vi "Launch as Nested Actor.vi"(6 "timeout in ms (-1)":i32=-1, 8 "Error In":errorcluster, 9 "Panel":refnum<class "Panel.lvclass">, 10 "Panel Actor in":refnum<class "Panel Actor.lvclass">, 11 "Caller Actor in":refnum<class "Actor.lvclass">) -> (0 "Error Out":errorcluster, 2 "Actor's Enqueuer":refnum<class "Message Enqueuer.lvclass">, 3 "Caller Actor out":refnum<class "Actor.lvclass">)   [LabVIEW 2023, in "Panel Actor.lvlib" / "Panel Actor.lvclass"]
doc: "Launches a root panel as a nested actor of a non-panel actor.\n\n<B>Caller Actor In:</B> Nested caller Actor \n<B>Panel Actor In:</B> Panel actor to launch as nested actor\n<B>Panel:</B> Panel to use in displaying nested actor\n<B>timeout in ms</B> Time to wait for the panel to initialize\n<B>Error In:</B> Describes error conditions that occur before this node runs.\n\n<B>Caller Actor In:</B> Nested caller Actor \n<B>Actor's Enqueuer:</B> Enqueuer for newly spawned actor\n<B>Error Out:</B> Contains error information.\n----\nPlease see the following web address for additional documentation and tutorial information:\nhttp://www.mooregoodideas.com/mgi-panel-manager/\n\nAuthor: Derek Trepanier\n\nCopyright (c) 2018, Moore Good Ideas, Inc.\n\nAll rights reserved.\n\nRedistribution and use in source and binary forms, with or without modification, are permitted provided that the following conditions are met:\n\n * Redistributions of source code must retain the above copyright notice, this list of conditions and the following disclaimer.\n * Redistributions in binary form must reproduce the above copyright notice, this list of conditions and the following disclaimer in the documentation and/or other materials provided with the distribution.\n * Neither the name of Moore Good Ideas, Inc. nor the names of its contributors may be used to endorse or promote products derived from this software without specific prior written permission.\n\nTHIS SOFTWARE IS PROVIDED BY THE COPYRIGHT HOLDERS AND CONTRIBUTORS \"AS IS\" AND ANY EXPRESS OR IMPLIED WARRANTIES, INCLUDING, BUT NOT LIMITED TO, THE IMPLIED WARRANTIES OF MERCHANTABILITY AND FITNESS FOR A PARTICULAR PURPOSE ARE DISCLAIMED. IN NO EVENT SHALL THE COPYRIGHT OWNER OR CONTRIBUTORS BE LIABLE FOR ANY DIRECT, INDIRECT, INCIDENTAL, SPECIAL, EXEMPLARY, OR CONSEQUENTIAL DAMAGES (INCLUDING, BUT NOT LIMITED TO, PROCUREMENT OF SUBSTITUTE GOODS OR SERVICES; LOSS OF USE, DATA, OR PROFITS; OR BUSINESS INTERRUPTION) HOWEVER CAUSED AND ON ANY THEORY OF LIABILITY, WHETHER IN CONTRACT, STRICT LIABILITY, OR TORT (INCLUDING NEGLIGENCE OR OTHERWISE) ARISING IN ANY WAY OUT OF THE USE OF THIS SOFTWARE, EVEN IF ADVISED OF THE POSSIBILITY OF SUCH DAMAGE."
uses:
  Library/Panel Actor.lvclass
  Panel/Panel/Panel.lvclass
  builds/Framework/Actor Framework.lvlibp/1abvi3w/vi.lib/ActorFramework/Message Enqueuer/Message Enqueuer.lvclass
  builds/Framework/Actor Framework.lvlibp/1abvi3w/vi.lib/ActorFramework/Actor/Actor.lvclass
  Panel/Panel/Panel.lvclass/Panel.ctl
  Library/Panel Actor.lvclass/Panel Actor.ctl
  Panel/Init Waiter/Init Waiter.vi
  Panel/Init Waiter/Init Waiter.lvclass
  C:/Users/Public/Documents/Development/builds/Framework/Actor Framework.lvlibp/1abvi3w/vi.lib/ActorFramework/Actor/Actor.lvclass
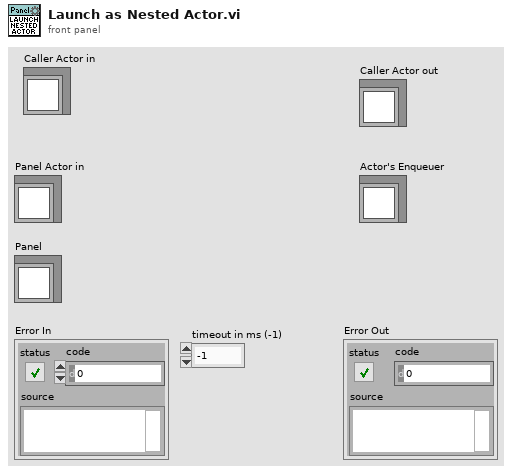
[diagram p1: front panel]
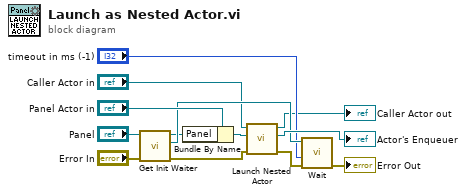
[diagram p0: block diagram]
diagram:
  n1 = call "Get Init Waiter.vi"("Error In"="Error In", "Panel In"="Panel") -> ("Error Out"=w8:errorcluster, "Init Waiter"=w7:refnum<class "Init Waiter.lvclass">, "Panel Out"=w1:refnum<class "Panel.lvclass">)  [unwired: 7 in]
  n2 = Bundle By Name(cluster="Panel Actor in", "Panel"=w1) -> (w12:refnum<class "Panel Actor.lvclass">)
  n3 = call "Launch Nested Actor.vi"("error in (no error)"=w8, "Nested Actor"=w12, "Caller Actor in"="Caller Actor in") -> ("error out"=w6:errorcluster, "Nested Actor's Enqueuer"=→"Actor's Enqueuer":refnum<class "Message Enqueuer.lvclass">, "Caller Actor out"=→"Caller Actor out":refnum<class "Actor.lvclass">)  [unwired: 6 in]
  n4 = call "Wait.vi"("Error In"=w6, "timeout in ms (-1)"="timeout in ms (-1)", "Init Waiter in"=w7) -> ("Error Out"=→"Error Out":errorcluster)  [unwired: 7 in, 1 out]
